vi "Global Error Strings.vi"() -> ()   [LabVIEW 2017, in "AB_Win_Common.lvlib"]
uses:
  <vilib>/InstallerBuilder/Common/AB_Win_Common.lvlib
panel:
  in  "Error.Source not top-level":string="The source type is not top-level."
  in  "Error.Source not found":string="Source not found."
  in  "Error.Shortcut not found":string="Shortcut not found."
  in  "Error.Registry value not found":string="Registry value not found."
  in  "Error.Install action not found":string="Install action not found."
  in  "Error.Product discovery":string="Error discovering products. A detailed log with more information can be found at \"%s.\""
  in  "Error.Duplicate shortcut":string="Shortcut \"%s\" associated with the file at \"%s\" and installed to \"%s\" has already been added."
  in  "Error.Duplicate registry value":string="Registry value \"%s\" at \"%s\" has already been added."
  in  "Warning.Product already included":string="Product \"%s\" already included."
  in  "Error.Product not found":string="Product \"%s\" not found."
  in  "Warning.Product already excluded":string="Product \"%s\" already excluded."
  in  "Error.Invalid registry location":string="Invalid registry location \"%s\". Registry hive \"%s\" not recognized."
  in  "Error.Default destination not found":string="Default destination \"%s\" was not found."
  in  "Error.Source file not found":string="Source file \"%s\" was not found."
  in  "Error.Shortcut ID not found":string="Shortcut ID \"%s\" was not found."
  in  "Error.Incorrect registry type":string="Registry value \"%s\" is of type \"%s,\" but expected type \"%s.\""
  in  "Error.Registry ID not found":string="Registry ID \"%s\" was not found."
  in  "Error.Unsupported source type":string="\"%s\" cannot be added because \"%s\" is not a supported type."
  in  "Error.Duplicate files":string="The following files were already added:\n%s"
  in  "Error.Cannot unlock paths":string="The following paths cannot be unlocked:\n%s"
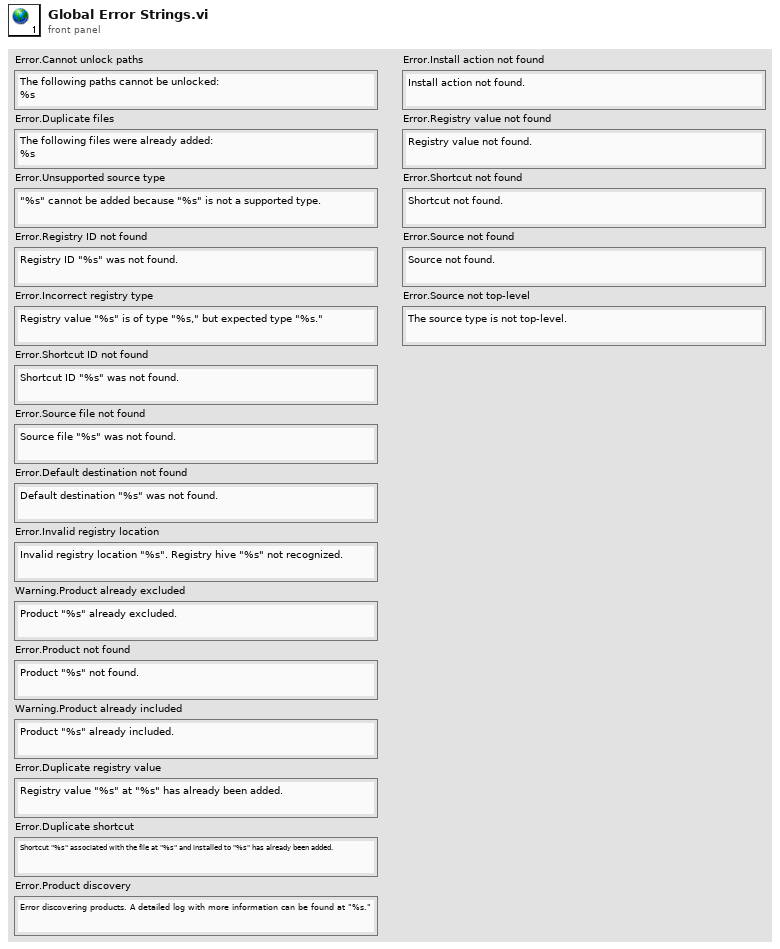
[diagram p1: front panel]
diagram:
